vi "Generate Event.vi"(4 "Actions":T2, 6 "Next State":T3, 7 "Act State":T3, 8 "Error In":errorcluster, 9 "Comment":string, 10 "Description":string, 11 "EventLog in":refnum<class "EventLog.lvclass">) -> (0 "Error Out":errorcluster, 3 "Events out":refnum<class "Events.lvclass">)   [LabVIEW 2019, in "Events.lvclass"]
uses:
  Events.lvclass
  Modules/Core/Core/TypeDef/App State.ctl
  SubModules/EventLog/EventLog.lvclass
  Modules/ModuleAbstract/ModuleAbstract/TypeDef/Module Actions.ctl
  <vilib>/ActorFramework/Message Enqueuer/Message Enqueuer.lvclass
  Events.lvclass/Events.ctl
  2c58f220-bd1a-47d2-9d68-2594ef47e403.vi
  9aa07609-5197-434a-a0da-376a16b3f738.vi
  <vilib>/Utility/Data Type/Get Numeric Information.vi
  Modules/Core/Core/Core.lvclass
  Modules/ModuleAbstract/ModuleAbstract/ModuleAbstract.lvclass
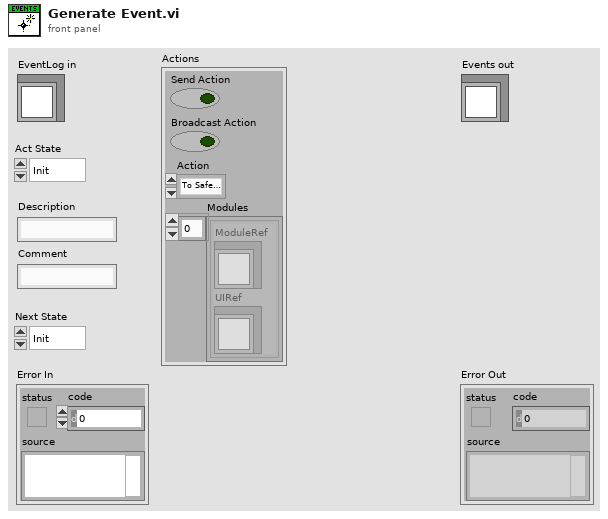
[diagram p1: front panel]
types:
  T1 = typedef "ModuleAbstract.lvlib/ModuleAbstract.lvclass/Module Actions.ctl" = enum16{"To Safe State", "Reset Safe State", "Close Module"}
  T2 = cluster{"Send Action":bool, "Broadcast Action":bool, "Action":T1, "Modules":cluster{"ModuleRef":refnum<class "Message Enqueuer.lvclass">, "UIRef":refnum<class "Message Enqueuer.lvclass">}[]}
  T3 = typedef "Core.lvlib/Core.lvclass/App State.ctl" = enum16{"Init", "Safe State", "Normal Working", "Closing"}
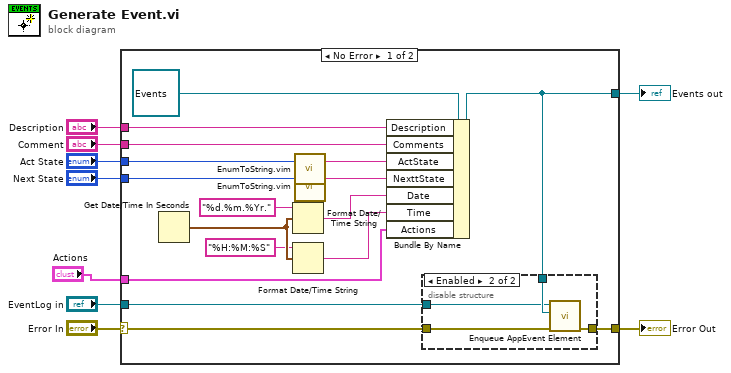
[diagram p0: block diagram]
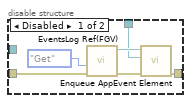
[diagram p2: hidden frame]
diagram:
  n1 = case shown="No Error" "Error In" {
    selector: "Error In" -> [w14 w37]
    tunnel: [w13 w37] -> w8
    tunnel: [w15 _] -> w7
    tunnel: "Description" -> [w26 _]
    tunnel: "Comment" -> [w25 _]
    tunnel: "Act State" -> [w24 _]
    tunnel: "Next State" -> [w23 _]
    tunnel: "EventLog in" -> [w12 _]
    tunnel: "Actions" -> [w10 _]
    frame No Error {
      n2 = Get Date/Time In Seconds() -> (seconds since 1Jan1904=w19:timestamp)
      n3 = Format Date/Time String(time format string (%c)="%d.%m.%Yr.", seconds (now)=w19) -> (date/time string=w17:string)  [unwired: 1 in]
      n4 = Format Date/Time String(time format string (%c)="%H:%M:%S", seconds (now)=w19) -> (date/time string=w16:string)  [unwired: 1 in]
      n5 = call "EnumToString.vim"("Enum"=w24) -> ("Enum Value"=w22:string)  [unwired: 16 in, 2 out]
      n6 = call "EnumToString.vim"("Enum"=w23) -> ("Enum Value"=w21:string)  [unwired: 16 in, 2 out]
      n7 = Bundle By Name(cluster=refnum<class "Events.lvclass"> refnum ("Events.lvclass"), "Description"=w26, "Comments"=w25, "ActState"=w22, "NexttState"=w21, "Date"=w17, "Time"=w16, "Actions"=w10) -> (w15:refnum<class "Events.lvclass">)
      n8 = disable-structure shown="Enabled" {
        disable-tunnel: w15 -> [w30 w34]
        disable-tunnel: w14 -> [w29 w35]
        disable-tunnel: [w28 w36] -> w13
        disable-tunnel: w12 -> [_ w33]
        frame Disabled {
          n9 = call "EventsLog Ref(FGV).vi"("Error In"=w29, "State"=enum16{"Get", "Set"}."Get") -> ("Error Out"=w31:errorcluster, "EventLog Out"=w32:refnum<class "EventLog.lvclass">)  [unwired: 8 in]
          n10 = call "Enqueue AppEvent Element.vi"("Error In"=w31, "Event Occured"=w30, "EventLog in"=w32) -> ("Error Out"=w28:errorcluster)  [unwired: 6 in, 2 out]
        }
        frame Enabled {
          n11 = call "Enqueue AppEvent Element.vi"("Error In"=w35, "Event Occured"=w34, "EventLog in"=w33) -> ("Error Out"=w36:errorcluster)  [unwired: 6 in, 2 out]
        }
      }
    }
    frame Error {
    }
  }
  "Error Out" <- w8
  "Events out" <- w7
